vi "TDMS Index File.vi"(8 "error in (no error)":errorcluster, 9 "Wait for Index to Complete? (F)":bool, 11 "TDMS File Path":path) -> (0 "error out":errorcluster, 3 "TDMS File Path Out":path)   [LabVIEW 2011]
uses:
  DIAdem/Datasheet/CGI Script Parameters.ctl
  DIAdem/Datasheet/Datasheet Generator Settings.ctl
  OpenG.LIB/file/file.llb/Convert File Extension (Path)__ogtk.vi
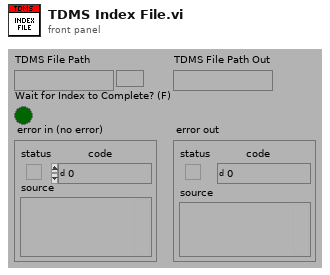
[diagram p1: front panel]
types:
  T1 = typedef "cgi Script parameters.ctl" = cluster{"Report Destination Path":path, "Script":string, "Total Parameters":dbl, "Parameter Names":string[], "Parameter Values":string[], "Scripts":string[], "Run Query?":bool}
  T2 = typedef "DATASHEET Generator Settings.ctl" = cluster{"Wait? (t)":bool, "ClientPrint? (f)":bool, "Client (\"\")":string, "joinPDF":bool, "Sort Method":enum16{"Item", "Template", "No Sort"}, "Export Row (-1=all)":i32, "Preview":bool, "Estimate Time":bool, "username":string, "jobid":string}
  T3 = typedef "CGI Script Parameters.ctl" = cluster{"Report Destination Path":path, "Script":string, "Total Parameters":dbl, "Parameter Names":string[], "Parameter Values":string[], "Scripts":string[], "Run Query?":bool}
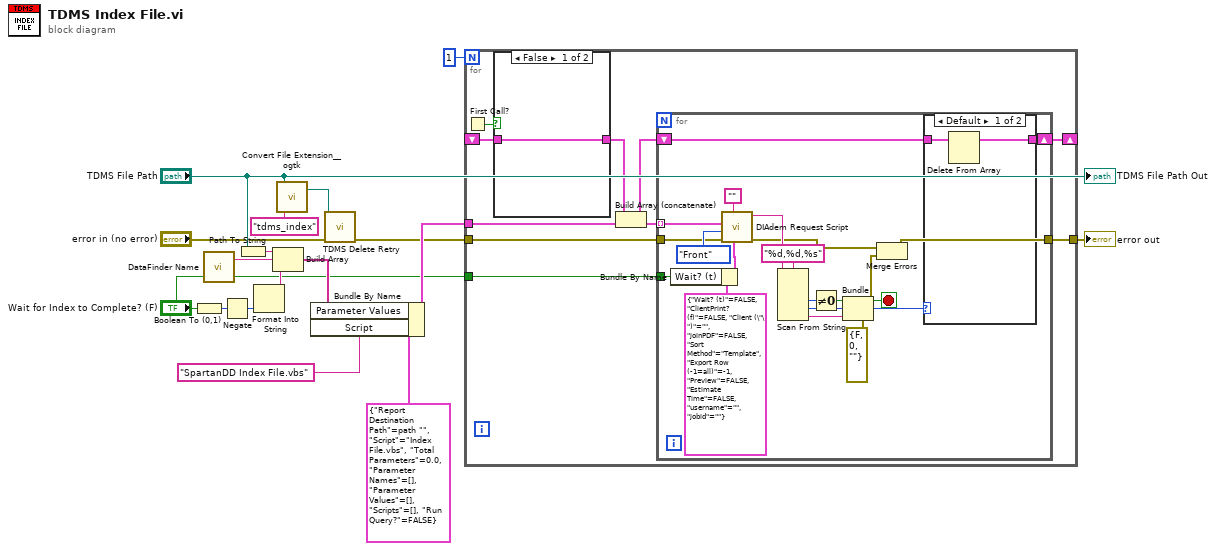
[diagram p0: block diagram]
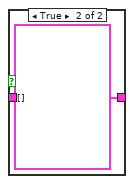
[diagram p3: hidden frame]
diagram:
  n1 = Boolean To (0,1)(Boolean="Wait for Index to Complete? (F)") -> (0, 1=w12:i16)
  n2 = call "DataFinder Name.vi"() -> ("DataFinder Name"=w7:string)  [unwired: 3 in]
  n3 = Negate(x=w12) -> (-x=w11:i16)
  n4 = Path To String(path="TDMS File Path") -> (string=w15:string)
  n5 = Format Into String(w11) -> (resulting string=w13:string)  [unwired: 3 in, 1 out]
  n6 = Build Array(w15, w7, w13) -> (w14:string[])
  n7 = call-poly "Convert File Extension__ogtk.vi"("new ending (none)"="tdms_index", "file name"="TDMS File Path") -> ("new filename"=w2:path)  [unwired: 1 out]
  n8 = Bundle By Name(cluster=T1 {"Report Destination Path"=path "", "Script"="Index File.vbs", "Total Parameters"=0.0, "Parameter Names"=[], "Parameter Values"=[], "Scripts"=[], "Run Query?"=FALSE} ("Script Parameters"), "Parameter Values"=w14, "Script"="SpartanDD Index File.vbs") -> (w16:T1)
  n9 = call "TDMS Delete Retry.vi"("error in"="error in (no error)", "path (use dialog)"=w2) -> ("error out"=w3:errorcluster)  [unwired: 9 out]
  n10 = for {
    N: 1 -> [_]
    tunnel: w16 -> [w21]
    tunnel: w3 -> [w26]
    tunnel: [w25] -> w10
    shift-right: [w19] -> _
    shift-left: _ -> [w23]
    tunnel: "Wait for Index to Complete? (F)" -> [w18]
    n11 = First Call?() -> (First Call?: T/F=w24:bool)
    n12 = case shown="False" w24 {
      tunnel: [w49 T3[] []] -> w22
      tunnel: w23 -> [w49 _]
      frame False {
      }
      frame True {
      }
    }
    n13 = Build Array (concatenate)(w22, w21) -> (w20:T1[])
    n14 = for {
      tunnel: w20 -> [w43] mode=indexing
      tunnel: w26 -> [w42]
      tunnel: [w27] -> w25
      shift-right: [w33] -> w19
      shift-left: w20 -> [w34]
      tunnel: w18 -> [w30]
      stop <- w37 stop-if-true
      n15 = Bundle By Name(cluster=T2 {"Wait? (t)"=FALSE, "ClientPrint? (f)"=FALSE, "Client (\"\")"="", "joinPDF"=FALSE, "Sort Method"=enum."Template", "Export Row (-1=all)"=-1, "Preview"=FALSE, "Estimate Time"=FALSE, "username"="", "jobid"=""} ("generator settings"), "Wait? (t)"=w30) -> (w31:T2)
      n16 = call "DIAdem Request Script.vi"("generator settings"=w31, "RunID"="", "error in (no error)"=w42, "Queue Entry"=enum16{"Front", "Back"}."Front", "Script Parameters"=w43) -> ("error out"=w28:errorcluster, "Result"=w41:string)  [unwired: 1 in, 4 out]
      n17 = Scan From String(format string="%d,%d,%s", input string=w41) -> (output 1=w39:i32, output 2=w36:i32, output 3=w35:string)  [unwired: 5 in, 3 out]
      n18 = Not Equal To 0?(x=w39) -> (x != 0?=w37:bool)
      n19 = Bundle(cluster=errorcluster {"status"=FALSE, "code"=0, "source"=""} ("error out"), "status"=w37, "code"=w36, "source"=w35) -> (w29:errorcluster)
      n20 = Merge Errors(w28, w29) -> (w27:errorcluster)
      n21 = case shown="Default" w36 {
        tunnel: w34 -> [w47 w48]
        tunnel: [w46 w48] -> w33
        frame Default {
          n22 = Delete From Array(array=w47) -> (array with subset deleted=w46:T1[])  [unwired: 2 in, 1 out]
        }
        frame -100101, -100100 {
          # "If there is an\nerror do to the\nDF having too\nmany items in its\nto-do list or\ntimeout, save\ntask and send\nagain next time\nthrough."
        }
      }
    }
  }
  "error out" <- w10
  "TDMS File Path Out" <- "TDMS File Path"
